vi "WFS Set Highspeed Mode.vi"(6 "Allow Auto Exposure (Off)":i32(ring) items=["On"=1, "Off"=0], 7 "Substract Offset":i32 format="%.0g", 8 "error in (no error)":errorcluster {"code" format="%.0x"}, 9 "Adapt Centroids (Off)":i32(ring) items=["On"=1, "Off"=0], 10 "Highspeed Mode (Off)":i32(ring) items=["On"=1, "Off"=0], 11 "instrument handle":refnum<visa-resource-name>) -> (0 "error out":errorcluster {"code" format="%.0x"}, 3 "instrument handle out":refnum<visa-resource-name>)   [LabVIEW 2020]
doc: "This VI activates/deactivates the camera's Highspeed Mode for WFS10/WFS20 instruments.\n\nWhen activated, the camera calculates the spot centroid positions internally and sends the result to the WFS driver instead of sending raw spotfield images.\n\nNote:\nThere is no camera image available when Highspeed Mode is activated!\nHighspeed Mode is not available for WFS150/WFS300/WFS30/WFS40 instruments!"
uses:
  WFS_32.dll
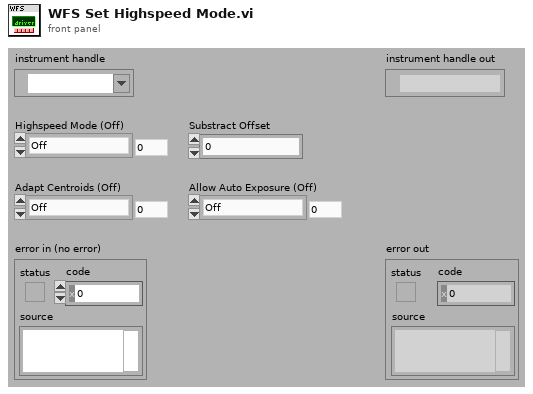
[diagram p1: front panel]
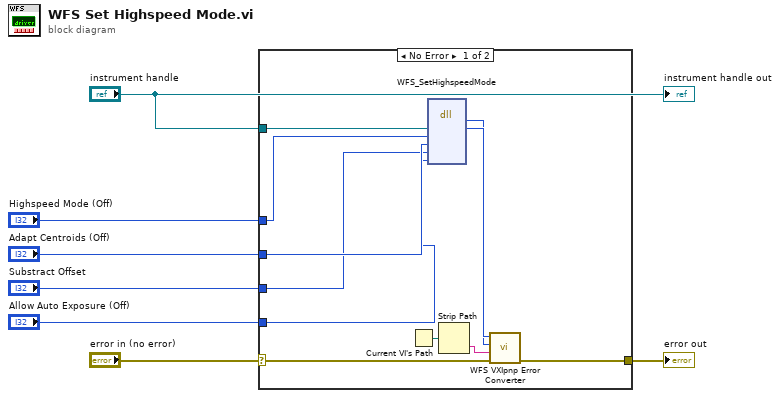
[diagram p0: block diagram]
diagram:
  n1 = case shown="No Error" "error in (no error)" {
    selector: "error in (no error)" -> [w13 w19]
    tunnel: [w12 w19] -> w7
    tunnel: "instrument handle" -> [w17 _]
    tunnel: "Highspeed Mode (Off)" -> [w11 _]
    tunnel: "Adapt Centroids (Off)" -> [w10 _]
    tunnel: "Substract Offset" -> [w9 _]
    tunnel: "Allow Auto Exposure (Off)" -> [w8 _]
    frame No Error {
      n2 = Current VI's Path() -> (path=w18:path)
      n3 = dll-call lib="WFS_*.*" fn="WFS_SetHighspeedMode"("Instrument Handle"=w17, "Highspeed Mode"=w11, "Adapt Centroids"=w10, "Substract Offset"=w9, "Allow Auto Exposure"=w8) -> (w15:i32, "Instrument Handle"=w16:u32)  [unwired: 7 in, 2 out]
      n4 = Strip Path(path=w18) -> (name=w14:string)  [unwired: 1 out]
      n5 = call "WFS VXIpnp Error Converter.vi"("error in (no error)"=w13, "Name Of VI (\"\")"=w14, "CVI Error Code (0)"=w15, "instrument handle"=w16) -> ("error out"=w12:errorcluster)  [unwired: 6 in, 1 out]
    }
    frame Error {
    }
  }
  "error out" <- w7
  "instrument handle out" <- "instrument handle"
